vi "Symphony Setup.vi"(4 "areas :":i32[][](array[numeric])=[[1], [1], [1], [1024], [256], [1], [1]], 6 "Acq type":i32(ring)=1 items=["JYMCD_ACQ_FORMAT_IMAGE", "JYMCD_ACQ_FORMAT_SCAN"], 7 "Int_time(ms)":i16=10 caption="Integration time(ms)", 8 "error in (no error)":errorcluster, 9 "Gain":i32, 10 "Select ADC":i32(ring) items=["JY_ADC_16_BIT", "JY_ADC_14_BIT", "JY_ADC_18_BIT"], 11 "JYCCDLib.IJYCCDReqd":refnum<k7>) -> (0 "error out":errorcluster, 1 "DataSize":i32, 3 "JYCCDLib.IJYCCDReqdOut":refnum<k7>)   [LabVIEW 2012]
panel:
  # "Area#"
  # "X Origin"
  # "Y Origin"
  # "X Size"
  # "Y Size"
  # "X Bin"
  # "Y Bin"
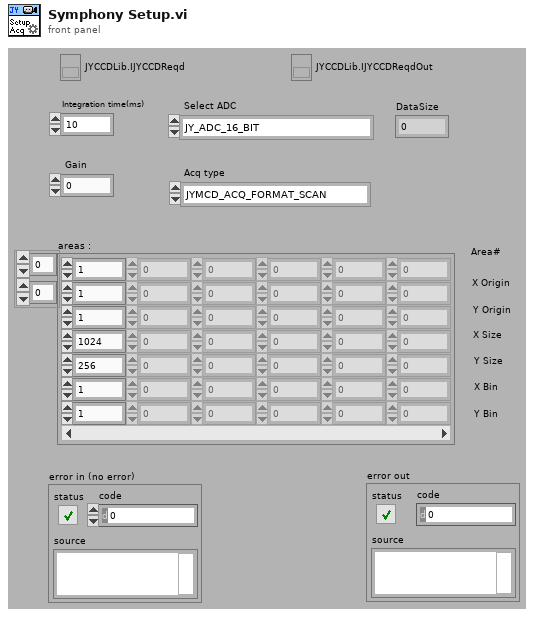
[diagram p1: front panel]
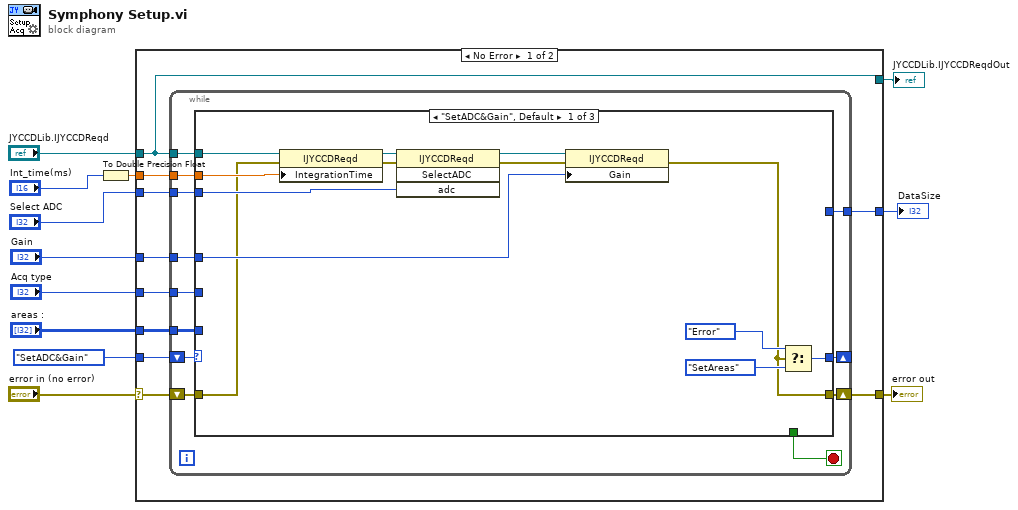
[diagram p0: block diagram]
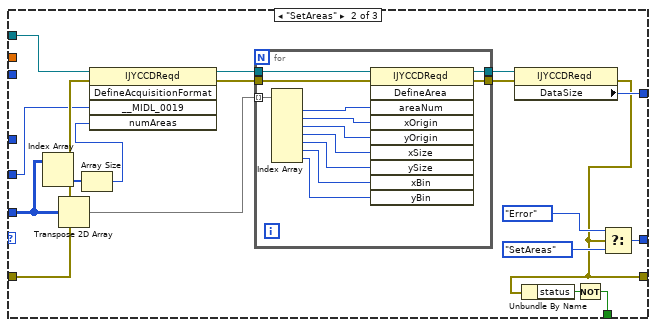
[diagram p2: hidden frame]
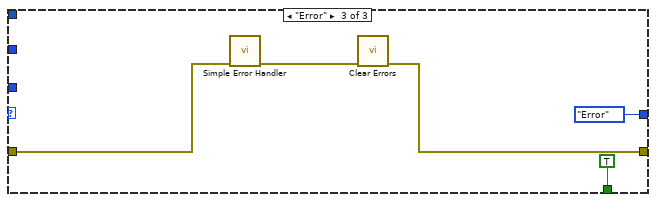
[diagram p3: hidden frame]
diagram:
  n1 = To Double Precision Float(number="Int_time(ms)") -> (double precision float=w7:dbl)
  n2 = case shown="No Error" "error in (no error)" {
    selector: "error in (no error)" -> [w22 w84]
    tunnel: [w21 w84] -> w11
    tunnel: enum16{"SetADC&Gain", "SetAreas", "Error"}."SetADC&Gain" -> [w20 _]
    tunnel: "JYCCDLib.IJYCCDReqd" -> [w17 w83]
    tunnel: w7 -> [w19 _]
    tunnel: "Select ADC" -> [w18 _]
    tunnel: [w17 w83] -> w5
    tunnel: "Gain" -> [w16 _]
    tunnel: "Acq type" -> [w15 _]
    tunnel: "areas :" -> [w14 _]
    tunnel: [w13 _] -> w1
    frame No Error {
      n3 = while {
        shift-right: [w29] -> w21
        shift-left: w22 -> [w32]
        tunnel: w17 -> [w33]
        shift-right: [w25] -> _
        shift-left: w20 -> [w34]
        tunnel: w19 -> [w31]
        tunnel: w18 -> [w30]
        tunnel: w16 -> [w28]
        tunnel: w15 -> [w27]
        tunnel: w14 -> [w26]
        tunnel: [w23] -> w13
        stop <- w24 stop-if-true
        n4 = case shown="\"SetADC&Gain\", Default" w34 {
          tunnel: w33 -> [w43 w52 _]
          tunnel: w32 -> [w35 w53 w82]
          tunnel: w31 -> [w42 _ _]
          tunnel: w30 -> [w41 _ _]
          tunnel: [w36 w56 w78] -> w29
          tunnel: w28 -> [w40 _ _]
          tunnel: w27 -> [_ w49 _]
          tunnel: w26 -> [_ w50 _]
          tunnel: [w37 w60 enum16{"SetADC&Gain", "SetAreas", "Error"}."Error"] -> w25
          tunnel: [_ w58 TRUE] -> w24
          tunnel: [_ w57 _] -> w23
          frame "SetADC&Gain", Default {
            n5 = property class="IJYCCDReqd"(reference=w43, error in=w35, "IntegrationTime"=w42) -> (reference out=w46:refnum<k7>, error out=w44:errorcluster)
            n6 = invoke class="IJYCCDReqd" method="SelectADC"(reference=w46, error in=w44, "adc"=w41) -> (reference out=w47:refnum<k7>, error out=w45:errorcluster)  [unwired: 1 in, 2 out]
            n7 = property class="IJYCCDReqd"(reference=w47, error in=w45, "Gain"=w40) -> (error out=w36:errorcluster)  [unwired: 1 out]
            n8 = Select(t=enum16{"SetADC&Gain", "SetAreas", "Error"}."Error", s=w36, f=enum16{"SetADC&Gain", "SetAreas", "Error"}."SetAreas") -> (s? t:f=w37:enum16{"SetADC&Gain", "SetAreas", "Error"})
          }
          frame "SetAreas" {
            n9 = Index Array(array=w50) -> (element=w51:i32[])  [unwired: 2 in]
            n10 = Transpose 2D Array(2D array=w50) -> (transposed array=w65:i32[][])
            n11 = Array Size(array=w51) -> (size(s)=w48:i32)
            n12 = invoke class="IJYCCDReqd" method="DefineAcquisitionFormat"(reference=w52, error in=w53, "__MIDL_0019"=w49, "numAreas"=w48) -> (reference out=w54:refnum<k7>, error out=w55:errorcluster)  [unwired: 1 in, 3 out]
            n13 = for {
              tunnel: [w76] -> w63
              tunnel: [w75] -> w64
              tunnel: w65 -> [w74] mode=indexing
              tunnel: w55 -> [w67]
              tunnel: w54 -> [w66]
              n14 = Index Array(array=w74) -> (element #1=w77:i32, element #2=w73:i32, element #3=w72:i32, element #4=w71:i32, element #5=w70:i32, element #6=w69:i32, element #7=w68:i32)  [unwired: 7 in]
              n15 = invoke class="IJYCCDReqd" method="DefineArea"(reference=w66, error in=w67, "areaNum"=w77, "xOrigin"=w73, "yOrigin"=w72, "xSize"=w71, "ySize"=w70, "xBin"=w69, "yBin"=w68) -> (reference out=w76:refnum<k7>, error out=w75:errorcluster)  [unwired: 1 in, 8 out]
            }
            n16 = property class="IJYCCDReqd"(reference=w63, error in=w64) -> (error out=w56:errorcluster, "DataSize"=w57:i32)  [unwired: 1 out]
            n17 = Unbundle By Name(w56) -> ("status"=w59:bool)
            n18 = Not(x=w59) -> (.not. x?=w58:bool)
            n19 = Select(t=enum16{"SetADC&Gain", "SetAreas", "Error"}."Error", s=w56, f=enum16{"SetADC&Gain", "SetAreas", "Error"}."SetAreas") -> (s? t:f=w60:enum16{"SetADC&Gain", "SetAreas", "Error"})
          }
          frame "Error" {
            n20 = call <vilib>:"Simple Error Handler.vi"("error in (no error)"=w82) -> ("error out"=w81:errorcluster)  [unwired: 4 in, 4 out]
            n21 = call <vilib>:"Clear Errors.vi"("error in (no error)"=w81) -> ("error out"=w78:errorcluster)  [unwired: 6 in]
          }
        }
      }
    }
    frame Error {
    }
  }
  "DataSize" <- w1
  "JYCCDLib.IJYCCDReqdOut" <- w5
  "error out" <- w11
